vi "Bundle test data.vi"(5 "Outputs in":T1, 6 "End Time":timestamp, 7 "Test Time (s)":dbl[](array[numeric]), 8 "Diameter (mm) Array":dbl[](array[numeric]), 9 "PWM Signal":dbl[](array[numeric]), 10 "Force (V)":dbl[](array[numeric]), 11 "Force Setpoint (V)":dbl[](array[numeric])) -> (3 "Outputs out":T1)   [LabVIEW 2020]
uses:
  Controls/Outputs.ctl
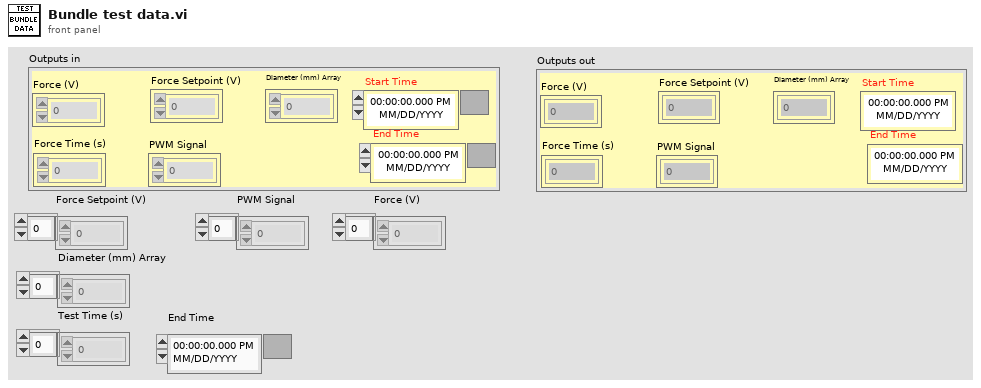
[diagram p1: front panel]
types:
  T1 = typedef "Outputs.ctl" = cluster{"Force Setpoint (V)":dbl[], "PWM Signal":dbl[], "Diameter (mm) Array":dbl[], "Force (V)":dbl[], "Force Time (s)":dbl[], "Start Time":timestamp, "End Time":timestamp}
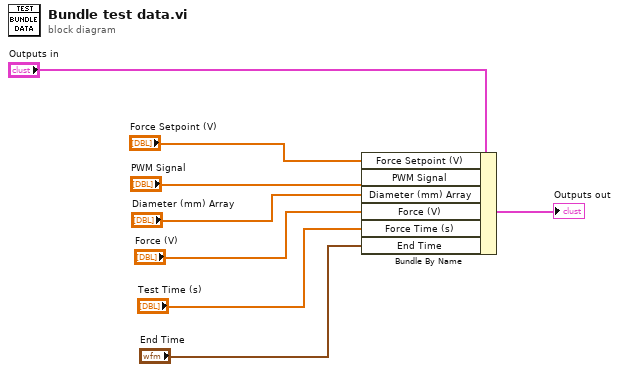
[diagram p0: block diagram]
diagram:
  n1 = Bundle By Name(cluster="Outputs in", "Force Setpoint (V)"="Force Setpoint (V)", "PWM Signal"="PWM Signal", "Diameter (mm) Array"="Diameter (mm) Array", "Force (V)"="Force (V)", "Force Time (s)"="Test Time (s)", "End Time"="End Time") -> (→"Outputs out":T1)
